vi "SP Read Array.vi"(8 "error in":errorcluster, 11 "Humidity Setpoint in":refnum<class "Humidity Setpoint.lvclass">) -> (0 "error out":errorcluster, 1 "Changed or First Call?":bool, 2 "Humidity SP":dbl[](array[numeric]), 3 "Humidity Setpoint out":refnum<class "Humidity Setpoint.lvclass">)   [LabVIEW 2023, in "Humidity Setpoint.lvclass"]
uses:
  Humidity Setpoint.lvclass
  Humidity Setpoint.lvclass/Humidity Setpoint.ctl
  Parents/Setpoint/Setpoint.lvclass
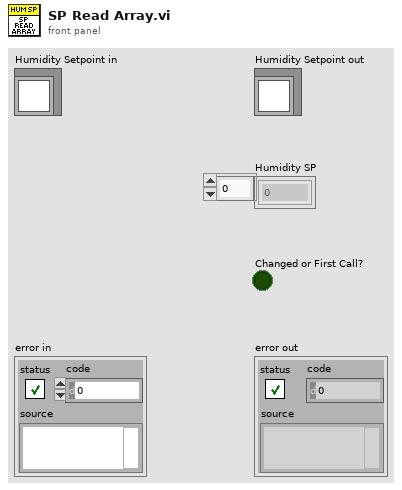
[diagram p1: front panel]
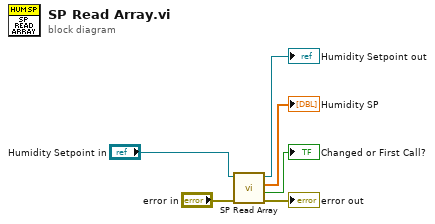
[diagram p0: block diagram]
diagram:
  n1 = call-parent "SP Read Array.vi"("error in"="error in", "Setpoint in"="Humidity Setpoint in") -> ("error out"=→"error out":errorcluster, "Changed or First Call?"=→"Changed or First Call?":bool, "Current Setpoint"=→"Humidity SP":dbl[], "Setpoint out"=→"Humidity Setpoint out":refnum<class "Humidity Setpoint.lvclass">)  [unwired: 6 in]
